vi "UWV_Analyse data_V1.0.vi"() -> ()   [LabVIEW 2015]
panel:
  out "Waveform Graph":dbl[][](graph)
  in  "record":i64
  out "# of records":i64
  in  "stop":bool
  in  "Record type":cluster{"Sampling rate":dbl, "Data":dbl[][]}
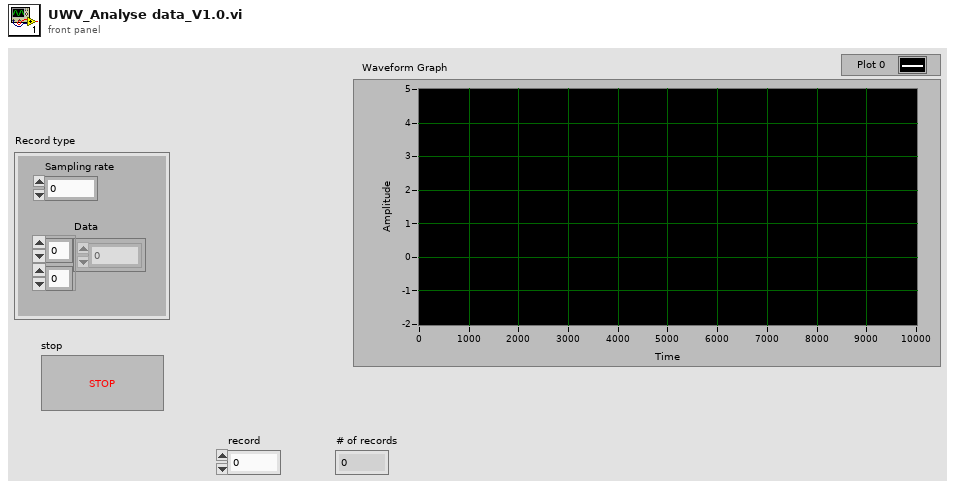
[diagram p1: front panel]
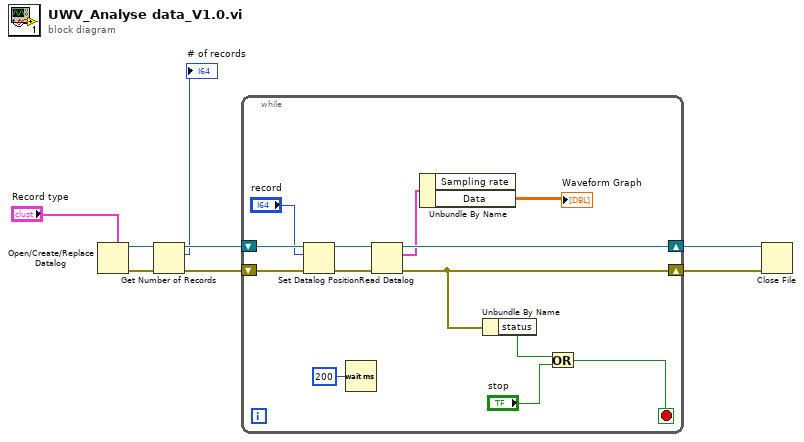
[diagram p0: block diagram]
diagram:
  n1 = Open/Create/Replace Datalog(5:"Record type") -> (0:w4:errorcluster, 3:w7:refnum<k1>)  [unwired: 5 in, 1 out]
  n2 = Get Number of Records(4:w4, 7:w7) -> (0:w3:errorcluster, 2:→"# of records":i64, 3:w6:refnum<k1>)
  n3 = while {
    shift-right: [w19] -> w5
    shift-left: w6 -> [w21]
    shift-right: [w12] -> w2
    shift-left: w3 -> [w18]
    stop <- w9 stop-if-true
    n4 = Set Datalog Position(4:w18, 6:"record", 7:w21) -> (0:w17:errorcluster, 3:w20:refnum<k1>)  [unwired: 1 in]
    n5 = Wait (ms)(milliseconds to wait=u32 200) -> ()  [unwired: 1 out]
    n6 = Read Datalog(4:w17, 7:w20) -> (0:w12:errorcluster, 2:w15:cluster{"Sampling rate":dbl, "Data":dbl[][]}, 3:w19:refnum<k1>)  [unwired: 1 in]
    n7 = Unbundle By Name(w15) -> ("Data"=→"Waveform Graph":dbl[][])  [unwired: 1 out]
    n8 = Unbundle By Name(w12) -> ("status"=w11:bool)
    n9 = Or(x=w11, y="stop") -> (x .or. y?=w9:bool)
  }
  n10 = Close File(refnum=w5, error in=w2) -> ()  [unwired: 2 out]
